vi "Emballage_BDD_Suppression_SQL_Cmd.vi"(8 "error in (no error)":errorcluster, 10 "NO_CDEVAL":string, 11 "Table (PRODUIT_EMBALLAGE)":string="PRODUIT_EMBALLAGE") -> (0 "error out":errorcluster)   [LabVIEW 2020]
uses:
  Modules/FS/60_FS_Controles/60_FS_SetGet.ctl
  <vilib>/addons/database/Connection.llb/DB Tools Open Connec (Path).vi
  <vilib>/addons/database/Connection.llb/Conn Execute.vi
  <vilib>/addons/database/Recordset.llb/Rec Destroy - Connection.vi
  <vilib>/addons/database/NI_Database_API.lvlib
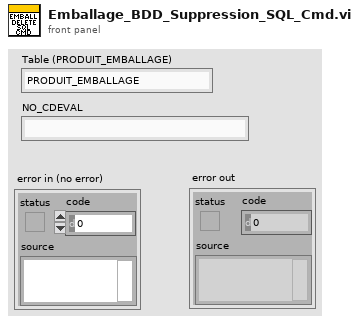
[diagram p1: front panel]
types:
  T1 = typedef "60_FS_SetGet.ctl" = enum16{"set", "get"}
  T2 = typedef "60_FS_CLT_Chemins.ctl" = cluster{"Racine_local":path, "Racine_reseau":path, "Racine_Support_Application":path, "Fichier_Journalisation":path, "Connexion_BDD_VSX":path, "Connexion_BDD_PLZ":path}
  T3 = typedef "NI_Database_API.lvlib/Conn ObjectReference.ctl" = refnum<k1>
  T4 = typedef "NI_Database_API.lvlib/Rec ObjectReference.ctl" = refnum<k1>
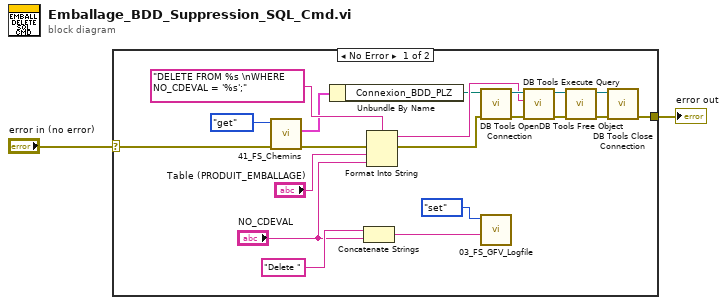
[diagram p0: block diagram]
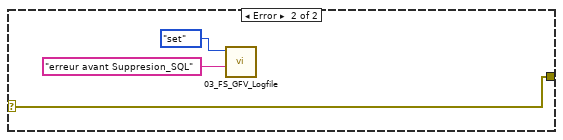
[diagram p2: hidden frame]
diagram:
  n1 = case shown="No Error" "error in (no error)" {
    selector: "error in (no error)" -> [w8 w25]
    tunnel: [w7 w25] -> w1
    frame No Error {
      n2 = call "41_FS_Chemins.vi"("error in (no error)"=w8, "SetGet"=60_FS_SetGet."get") -> ("error out"=w9:errorcluster, "CLT_Chemins_out"=w13:T2)  [unwired: 8 in]
      n3 = Unbundle By Name(w13) -> ("Connexion_BDD_PLZ"=w11:path)
      n4 = Concatenate Strings("Delete " ("chaîne"), "NO_CDEVAL") -> (w5:string)
      n5 = Format Into String(format string="DELETE FROM %s \nWHERE NO_CDEVAL = '%s';" ("chaîne de format"), error in=w9, "Table (PRODUIT_EMBALLAGE)", "NO_CDEVAL") -> (resulting string=w16:string, error out=w14:errorcluster)  [unwired: 1 in]
      n6 = call-poly <vilib>:"DB Tools Open Connection.vi"("error in (no error)"=w14, "connection information"=w11) -> ("error out"=w22:errorcluster, "connection reference"=w17:T3)  [unwired: 6 in]
      n7 = call "03_FS_GFV_Logfile.vi"("Chaîne"=w5, "States"=60_FS_SetGet."set") -> ()  [unwired: 8 in, 2 out]
      n8 = call-poly <vilib>:"DB Tools Execute Query.vi"("error in (no error)"=w22, "SQL query"=w16, "connection reference"=w17) -> ("error out"=w21:errorcluster, "recordset reference"=w20:T4)  [unwired: 5 in]
      n9 = call-poly <vilib>:"DB Tools Free Object.vi"("error in (no error)"=w21, "recordset reference"=w20) -> ("error out"=w19:errorcluster, "connection reference"=w18:T3)  [unwired: 8 in]
      n10 = call <vilib>:"DB Tools Close Connection.vi"("error in (no error)"=w19, "connection reference"=w18) -> ("error out"=w7:errorcluster)  [unwired: 5 in]
    }
    frame Error {
      n11 = call "03_FS_GFV_Logfile.vi"("Chaîne"="erreur avant Suppresion_SQL", "States"=60_FS_SetGet."set") -> ()  [unwired: 8 in, 2 out]
    }
  }
  "error out" <- w1
